vi "Errors.vi"   [LabVIEW 2017, in "DSF Core.lvlib" / "Configuration Session.lvclass"]
uses:
  Configuration Session.lvclass
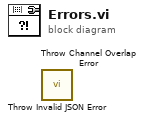
[diagram p0: block diagram]
diagram:
  n1 = call "Throw Invalid JSON Error.vi"() -> ()  [unwired: 11 in, 1 out]
  n2 = call "Throw Channel Overlap Error.vi"() -> ()  [unwired: 11 in, 1 out]
